vi "execute.vi"(8 "error in (no error)":errorcluster, 10 "Context in":refnum<class "Context.lvclass">, 11 "ApplyAberrationByForcesCommand in":refnum<class "ApplyAberrationByForcesCommand.lvclass">) -> (0 "error out":errorcluster, 2 "Context out":refnum<class "Context.lvclass">, 3 "ApplyAberrationByForcesCommand out":refnum<class "ApplyAberrationByForcesCommand.lvclass">)   [LabVIEW 2016, in "ApplyAberrationByForcesCommand.lvclass"]
uses:
  ApplyAberrationByForcesCommand.lvclass
  Context/Context.lvclass
  ApplyAberrationByForcesCommand.lvclass/ApplyAberrationByForcesCommand.ctl
  Context/Context.lvclass/Context.ctl
  Context/getModel.vi
  Context/setModel.vi
  Model/getState.vi
  States/State/State.lvclass
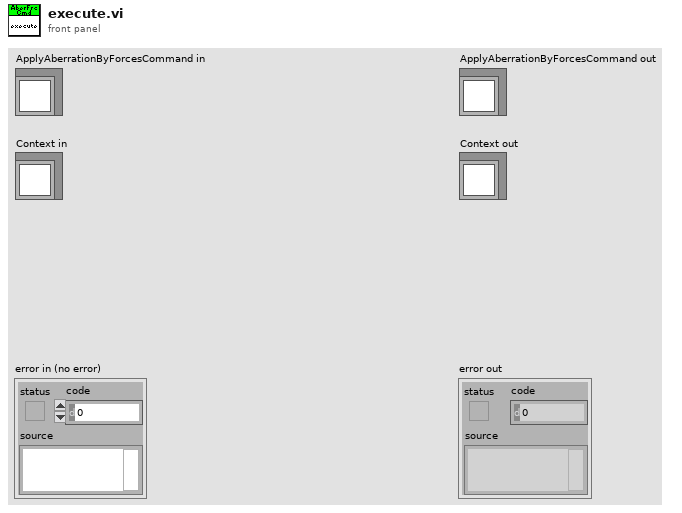
[diagram p1: front panel]
types:
  T1 = typedef "M1M3SupportTopics.lvlib/CommandApplyAberrationByForces.ctl" = cluster{"CommandId":T2, "ZForces":dbl[]}
  T2 = typedef "M1M3SupportTopics.lvlib/CommandId.ctl" = i32
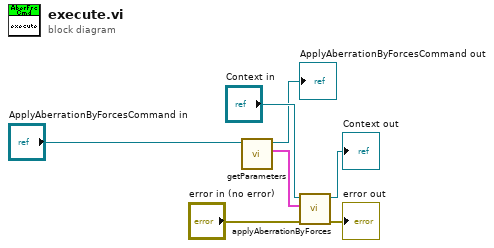
[diagram p0: block diagram]
diagram:
  n1 = call "getParameters.vi"("ApplyAberrationByForcesCommand in"="ApplyAberrationByForcesCommand in") -> ("Parameters"=w3:T1, "ApplyAberrationByForcesCommand out"=→"ApplyAberrationByForcesCommand out":refnum<class "ApplyAberrationByForcesCommand.lvclass">)  [unwired: 9 in]
  n2 = call "applyAberrationByForces.vi"("error in (no error)"="error in (no error)", "Parameters"=w3, "Context in"="Context in") -> ("error out"=→"error out":errorcluster, "Context out"=→"Context out":refnum<class "Context.lvclass">)  [unwired: 7 in]
